vi "Filtering - global gate.vi"(8 "error in (no error)":errorcluster) -> (0 "error out":errorcluster)   [LabVIEW 2026, in "Tests.lvlib"]
doc: "Integration test. Verifies that a single Log call fans out to every registered appender: registers three queue-mode relay appenders, logs one Info message, and asserts each appender's queue receives exactly one Statement with identical payload. Every gate except fan-out is held open (global threshold at floor, permissive filters, unbounded queues), so a missing element can only be a fan-out defect.\n\nImplements LMBR-T-030 -> SRS-019, SRS-028. Assert-level IDs: Test-ID-Assert-Checklist.md."
uses:
  Tests.lvlib
  src/TypeDefs/Severity.ctl
  <vilib>/addons/_JKI Toolkits/Caraya/classes/Assert/Assert Equal Value_Variant.vi
  <vilib>/addons/_JKI Toolkits/Caraya/classes/Assert/Assert True.vi
  <vilib>/addons/_JKI Toolkits/Caraya/classes/Test/Test.lvclass
  src/Lumberjack.lvlib
  src/Public/Logger.lvclass/Logger.lvclass
  <vilib>/addons/_JKI Toolkits/Caraya/classes/Assert/Assert.lvclass
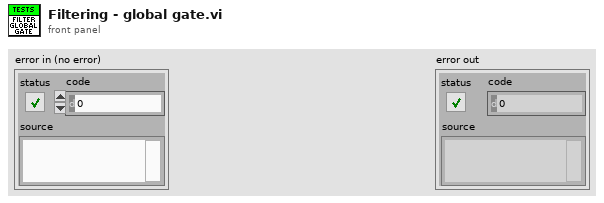
[diagram p1: front panel]
types:
  T1 = typedef "Lumberjack.lvlib/Severity.ctl" = enum16{"OFF", "FATAL", "ERROR", "WARN", "INFO", "DEBUG", "TRACE", "ALL"}
  T2 = typedef "Lumberjack.lvlib/Statement.ctl" = cluster{"timestamp":timestamp, "level":T1, "sourceTag":string, "originVI":string, "message":string}
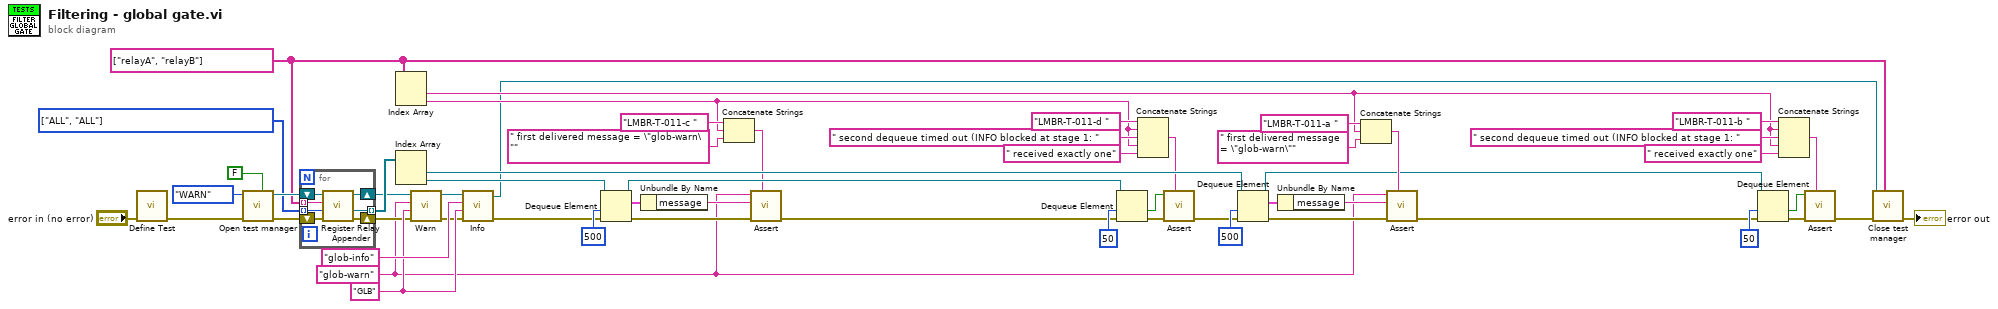
[diagram p0: block diagram]
diagram:
  w1 = "glob-warn" ("message")
  w49 = T1[] [enum."ALL", enum."ALL"] items=["OFF", "FATAL", "ERROR", "WARN", "INFO", "DEBUG", "TRACE", "ALL"]
  w48 = "GLB" ("sourceTag")
  w11 = string[] ["relayA", "relayB"]
  n1 = call <vilib>:"Define Test.vi"("error in (no error)"="error in (no error)") -> ("error out"=w56:errorcluster)  [unwired: 9 in, 1 out]
  n2 = call "Open test manager.vi"("enableDefaultFile"=FALSE, "error in (no error)"=w56, "globalThreshold"=Severity."WARN") -> ("error out"=w52:errorcluster, "Logger out"=w53:refnum<class "Logger.lvclass">)  [unwired: 7 in]
  n3 = for {
    shift-right: [w62] -> w8
    shift-left: w53 -> [w64]
    shift-right: [w61] -> w6
    shift-left: w52 -> [w63]
    tunnel: w11 -> [w60] mode=indexing
    tunnel: [w59] -> w47 mode=indexing
    tunnel: w49 -> [w58] mode=indexing
    n4 = call "Register Relay Appender.vi"("error in (no error)"=w63, "threshold"=w58, "id in"=w60, "Logger in"=w64) -> ("error out"=w61:errorcluster, "relayQueue"=w59:refnum<queue>, "Logger out"=w62:refnum<class "Logger.lvclass">)  [unwired: 4 in, 1 out]
  }
  n5 = Index Array(array=w11) -> (element #1=w32:string, element #2=w12:string)  [unwired: 2 in]
  n6 = Index Array(array=w47) -> (element #1=w40:refnum<queue>, element #2=w13:refnum<queue>)  [unwired: 2 in]
  n7 = call "Warn.vi"("error in (no error)"=w6, "sourceTag"=w48, "message"=w1, "Logger in"=w8) -> ("error out"=w5:errorcluster, "Logger out"=w7:refnum<class "Logger.lvclass">)  [unwired: 6 in]
  n8 = call "Info.vi"("error in (no error)"=w5, "sourceTag"=w48, "message"="glob-info", "Logger in"=w7) -> ("error out"=w4:errorcluster, "Logger out"=w9:refnum<class "Logger.lvclass">)  [unwired: 6 in]
  n9 = Dequeue Element(queue=w13, timeout in ms (-1)=500, error in (no error)=w4) -> (queue out=w23:refnum<queue>, element=w26:T2, error out=w24:errorcluster)  [unwired: 1 out]
  n10 = Unbundle By Name(w26) -> ("message"=w25:string)
  n11 = Concatenate Strings("LMBR-T-011-c ", w12, " first delivered message = \"glob-warn\"") -> (w15:string)
  n12 = call-poly <vilib>:"Assert.vi"("Label"=w15, "error in (no error)"=w24, "Actual"=w25, "Expected"=w1) -> ("error out"=w22:errorcluster)  [unwired: 6 in, 1 out]
  n13 = Dequeue Element(queue=w23, timeout in ms (-1)=50, error in (no error)=w22) -> (timed out?=w28:bool, error out=w29:errorcluster)  [unwired: 2 out]
  n14 = Concatenate Strings("LMBR-T-011-d ", w12, " second dequeue timed out (INFO blocked at stage 1: ", w12, " received exactly one") -> (w16:string)
  n15 = call-poly <vilib>:"Assert.vi"("Label"=w16, "error in (no error)"=w29, "True?"=w28) -> ("error out"=w14:errorcluster)  [unwired: 7 in, 1 out]
  n16 = Dequeue Element(queue=w40, timeout in ms (-1)=500, error in (no error)=w14) -> (queue out=w2:refnum<queue>, element=w45:T2, error out=w39:errorcluster)  [unwired: 1 out]
  n17 = Unbundle By Name(w45) -> ("message"=w44:string)
  n18 = Concatenate Strings("LMBR-T-011-a ", w32, " first delivered message = \"glob-warn\"") -> (w31:string)
  n19 = call-poly <vilib>:"Assert.vi"("Label"=w31, "error in (no error)"=w39, "Actual"=w44, "Expected"=w1) -> ("error out"=w3:errorcluster)  [unwired: 6 in, 1 out]
  n20 = Dequeue Element(queue=w2, timeout in ms (-1)=50, error in (no error)=w3) -> (timed out?=w41:bool, error out=w42:errorcluster)  [unwired: 2 out]
  n21 = Concatenate Strings("LMBR-T-011-b ", w32, " second dequeue timed out (INFO blocked at stage 1: ", w32, " received exactly one") -> (w33:string)
  n22 = call-poly <vilib>:"Assert.vi"("Label"=w33, "error in (no error)"=w42, "True?"=w41) -> ("error out"=w50:errorcluster)  [unwired: 7 in, 1 out]
  n23 = call "Close test manager.vi"("queueIDList"=w11, "error in (no error)"=w50, "Logger in"=w9) -> ("error out"=→"error out":errorcluster)  [unwired: 6 in]
